vi "Multiline String to 1D String Array.vi"(0 "Multiline Input String":string, 1 "Number of Elements":i16) -> (2 "1D String Output Array":string[](array[string]))   [LabVIEW 2024]
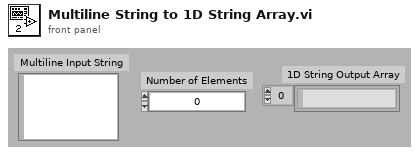
[diagram p1: front panel]
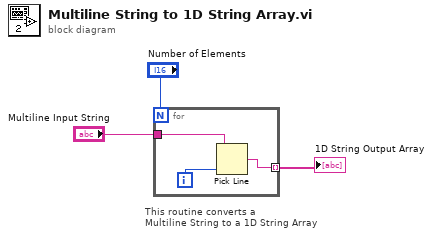
[diagram p0: block diagram]
diagram:
  n1 = for "This routine converts a\nMultiline String to a 1D String Array" {
    N: "Number of Elements" -> [_]
    tunnel: "Multiline Input String" -> [w5]
    tunnel: [w4] -> w1 mode=indexing
    i -> [w6]
    n2 = Pick Line(multi-line string=w5, line index=w6) -> (output string=w4:string)  [unwired: 1 in]
  }
  "1D String Output Array" <- w1
